vi "I16.vi"(1 "Numeric Input":i16) -> (0 "Numeric Output":i16)   [LabVIEW 2011]
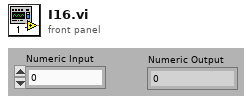
[diagram p1: front panel]
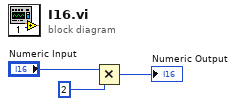
[diagram p0: block diagram]
diagram:
  n1 = Multiply(x="Numeric Input", y=i16 2) -> (x*y=→"Numeric Output":i16)
